vi "Scan lines to grid area.vi"(5 "Enable":bool, 6 "Grid settings":T1, 7 "Multilines":u16, 8 "Y line in":u32, 9 "Y scan line":u32, 10 "Multi-line scan":i16[](array[numeric]), 11 "Input array":i16[][][][](array[numeric])) -> (0 "Y line out":u32, 3 "Ouput array":i16[][][][](array[numeric]))   [LabVIEW 2018]
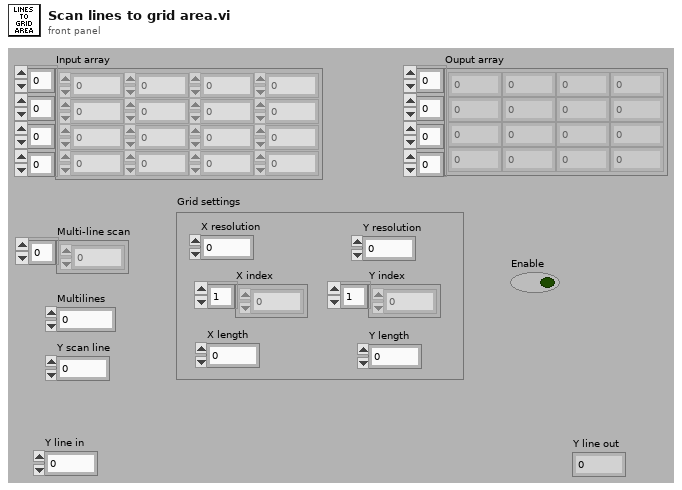
[diagram p1: front panel]
types:
  T1 = cluster{"X resolution":u32, "Y resolution":u32, "X index":u32[], "Y index":u32[], "X length":u32, "Y length":u32}
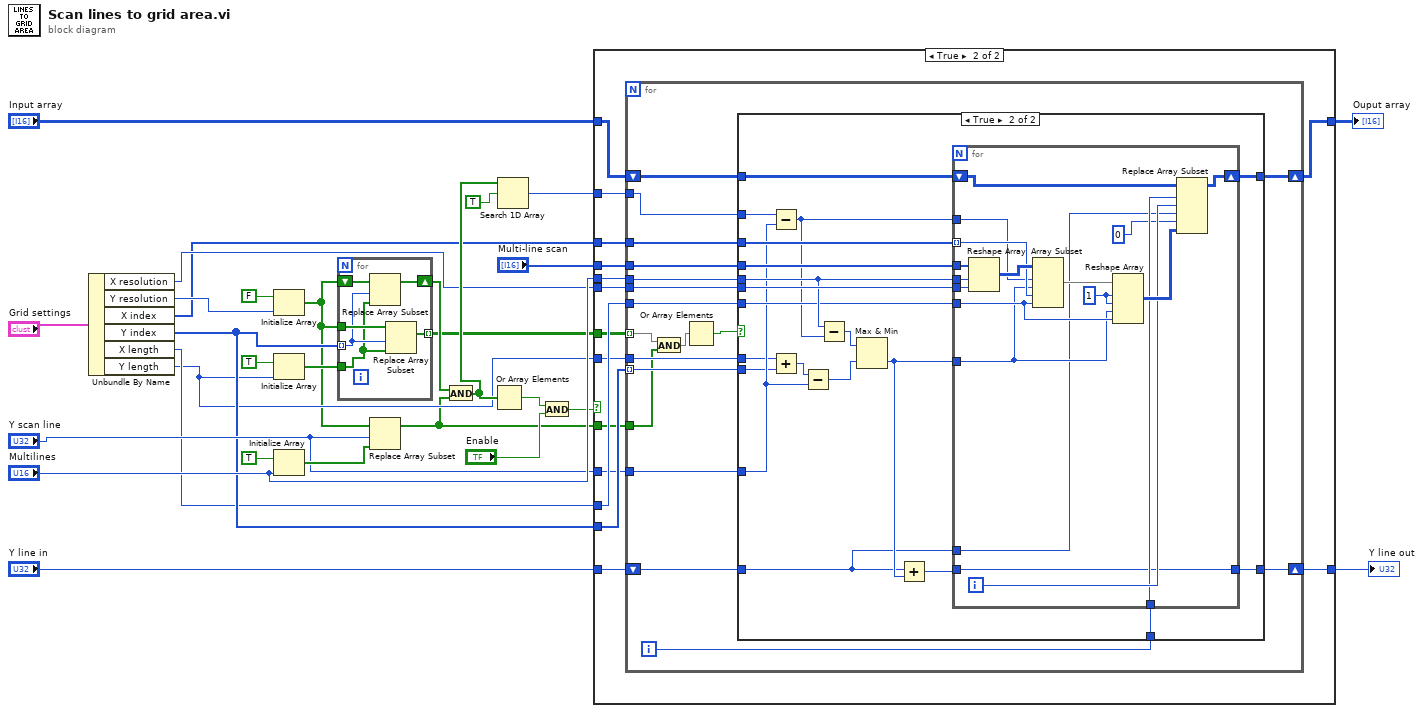
[diagram p0: block diagram]
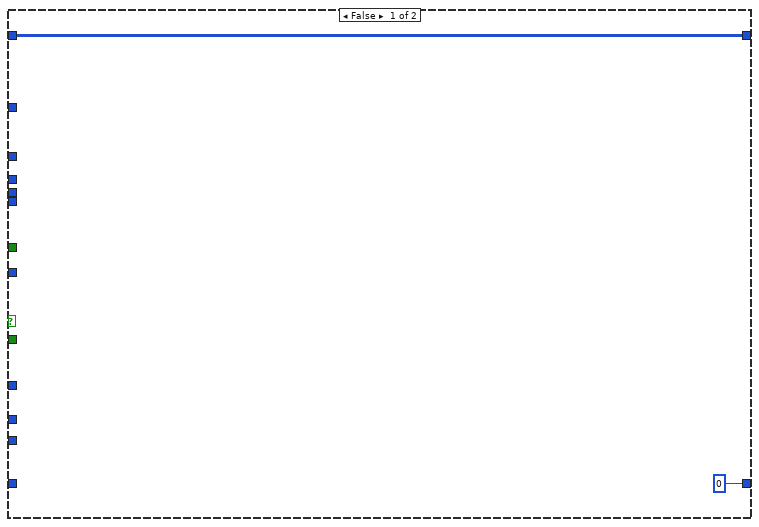
[diagram p2: hidden frame]
diagram:
  n1 = Unbundle By Name("Grid settings") -> ("X resolution"=w8:u32, "Y resolution"=w10:u32, "X index"=w7:u32[], "Y index"=w9:u32[], "X length"=w6:u32, "Y length"=w5:u32)
  n2 = Initialize Array(FALSE ("element"), w10) -> (w1:bool[])
  n3 = Initialize Array(TRUE ("element"), w5) -> (w29:bool[])
  n4 = Initialize Array(TRUE ("element"), "Multilines") -> (w24:bool[])
  n5 = for {
    tunnel: w9 -> [w31] mode=indexing
    shift-right: [w34] -> w26
    shift-left: w1 -> [w35]
    tunnel: w29 -> [w30]
    tunnel: [w32] -> w3 mode=indexing
    tunnel: w1 -> [w33]
    n6 = Replace Array Subset(array=w35, new element=w30, index=w31) -> (w34:bool[])
    n7 = Replace Array Subset(array=w33, new element=w30, index=w31) -> (w32:bool[])
  }
  n8 = Replace Array Subset(array=w1, new element=w24, index="Y scan line") -> (w2:bool[])
  n9 = And(x=w26, y=w2) -> (x .and. y?=w15:bool[])
  n10 = Or Array Elements(Boolean array=w15) -> (logical OR=w19:bool)
  n11 = Search 1D Array(1D array=w15, element=TRUE) -> (index of element=w16:i32)  [unwired: 1 in]
  n12 = And(x=w19, y="Enable") -> (x .and. y?=w18:bool)
  n13 = case shown="True" w18 {
    tunnel: "Input array" -> [w37 w51]
    tunnel: w7 -> [_ w52]
    tunnel: [w37 w50] -> w22
    tunnel: "Multi-line scan" -> [_ w49]
    tunnel: w8 -> [_ w48]
    tunnel: "Multilines" -> [_ w47]
    tunnel: w6 -> [_ w46]
    tunnel: w16 -> [_ w45]
    tunnel: w9 -> [_ w44]
    tunnel: "Y scan line" -> [_ w43]
    tunnel: w5 -> [_ w42]
    tunnel: "Y line in" -> [_ w41]
    tunnel: [u32 0 ("Y line in") w40] -> w12
    tunnel: w3 -> [_ w39]
    tunnel: w2 -> [_ w38]
    frame False {
    }
    frame True {
      n14 = for {
        tunnel: w52 -> [w70]
        shift-right: [w68] -> w50
        shift-left: w51 -> [w69]
        tunnel: w49 -> [w67]
        tunnel: w48 -> [w66]
        tunnel: w47 -> [w65]
        tunnel: w46 -> [w64]
        tunnel: w45 -> [w59]
        tunnel: w44 -> [w61] mode=indexing
        tunnel: w43 -> [w63]
        tunnel: w42 -> [w60]
        shift-right: [w58] -> w40
        shift-left: w41 -> [w57]
        tunnel: w39 -> [w54] mode=indexing
        tunnel: w38 -> [w53]
        i -> [w62]
        n15 = And(x=w54, y=w53) -> (x .and. y?=w56:bool[])
        n16 = Or Array Elements(Boolean array=w56) -> (logical OR=w55:bool)
        n17 = case shown="True" w55 {
          tunnel: w70 -> [_ w92]
          tunnel: w69 -> [w72 w91]
          tunnel: [w72 w90] -> w68
          tunnel: w67 -> [_ w89]
          tunnel: w66 -> [_ w88]
          tunnel: w65 -> [_ w87]
          tunnel: w64 -> [_ w86]
          tunnel: w63 -> [_ w85]
          tunnel: w62 -> [_ w84]
          tunnel: w61 -> [_ w82]
          tunnel: w60 -> [_ w81]
          tunnel: w59 -> [_ w77]
          tunnel: [w71 w74] -> w58
          tunnel: w57 -> [w71 w73]
          frame False {
          }
          frame True {
            n18 = Subtract(x=w77, y=w85) -> (x-y=w76:u32)
            n19 = Add(x=w81, y=w82) -> (x+y=w83:u32)
            n20 = Subtract(x=w83, y=w85) -> (x-y=w80:u32)
            n21 = Subtract(x=w87, y=w76) -> (x-y=w79:u32)
            n22 = Max & Min(x=w79, y=w80) -> (min(x,y)=w78:u32)  [unwired: 1 out]
            n23 = Add(x=w73, y=w78) -> (x+y=w75:u32)
            n24 = for {
              tunnel: w92 -> [w104] mode=indexing
              shift-right: [w109] -> w90
              shift-left: w91 -> [w110]
              tunnel: w89 -> [w107]
              tunnel: w88 -> [w106]
              tunnel: w87 -> [w105]
              tunnel: w86 -> [w100]
              tunnel: w84 -> [w96]
              tunnel: w78 -> [w98]
              tunnel: w76 -> [w97]
              tunnel: w75 -> [w95]
              tunnel: [w95] -> w74
              tunnel: w73 -> [w94]
              i -> [w99]
              w101 = 1 ("dimension size")
              n25 = Reshape Array(w107, w105, w106) -> (w108:i16[][])
              n26 = Array Subset(array=w108, index (row)=w97, length (row)=w98, index (col)=w104, length (col)=w100) -> (w103:i16[][])
              n27 = Reshape Array(w103, w101, w101, w98, w100) -> (w102:i16[][][][])
              n28 = Replace Array Subset(array=w110, new element=w102, index (dim 0)=w96, index (dim 1)=w99, index (dim 2)=w94, index (dim 3)=0 ("index (col)")) -> (w109:i16[][][][])
            }
          }
        }
      }
    }
  }
  "Ouput array" <- w22
  "Y line out" <- w12
